vi "Close.vi"(8 "Error In":errorcluster, 11 "SDO Manager":refnum<class "SDO Manager.lvclass">) -> (0 "Error Out":errorcluster, 3 "SDO Manager":refnum<class "SDO Manager.lvclass">)   [LabVIEW 2020, in "CANopen.lvlib" / "SDO Manager.lvlib" / "SDO Manager.lvclass"]
uses:
  SDO Manager.lvclass
  SDO Manager.lvclass/SDO Manager.ctl
  <vilib>/ActorFramework/Stop Msg/Stop Msg.lvclass
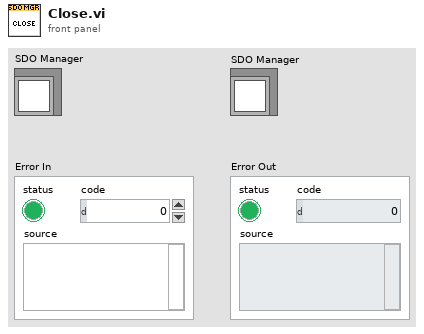
[diagram p1: front panel]
types:
  T1 = map{u8, refnum<class "Message Enqueuer.lvclass">}
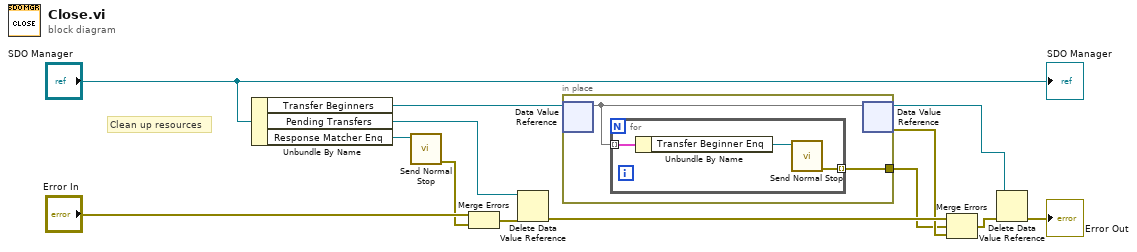
[diagram p0: block diagram]
diagram:
  # "Clean up resources"
  n1 = Unbundle By Name("SDO Manager") -> ("Transfer Beginners"=w5:refnum<data-value>, "Pending Transfers"=w6:refnum<data-value>, "Response Matcher Enq"=w12:refnum<class "Message Enqueuer.lvclass">)
  n2 = call <vilib>:"Send Normal Stop.vi"("Message Enqueuer"=w12) -> ("error out"=w8:errorcluster)  [unwired: 10 in]
  n3 = Merge Errors("Error In", w8) -> (w10:errorcluster)
  n4 = Delete Data Value Reference(data value reference=w6, error in=w10) -> (error out=w11:errorcluster)  [unwired: 1 out]
  n5 = in-place {
    in-place-border: [w15] -> w1
    n6 = in-place-dvr #1(w5) -> (w14:T1)  [unwired: 1 out]
    n7 = for {
      tunnel: w14 -> [w18] mode=indexing
      tunnel: [w16] -> w15 mode=indexing
      n8 = Unbundle By Name(w18) -> ("Transfer Beginner Enq"=w17:refnum<class "Message Enqueuer.lvclass">)
      n9 = call <vilib>:"Send Normal Stop.vi"("Message Enqueuer"=w17) -> ("error out"=w16:errorcluster)  [unwired: 10 in]
    }
    n10 = in-place-dvr #1(w14) -> (w4:refnum<data-value>, w2:errorcluster)
  }
  n11 = Merge Errors(w11, w1, w2) -> (w3:errorcluster)
  n12 = Delete Data Value Reference(data value reference=w4, error in=w3) -> (error out=→"Error Out":errorcluster)  [unwired: 1 out]
  "SDO Manager" <- "SDO Manager"
